vi "Inst_Nexus.vi"(8 "error in":errorcluster, 10 "All Message Queues in":T1, 11 "AjustesPrevios in":refnum<class "AjustesPrevios.lvclass">) -> (0 "error out":errorcluster)   [LabVIEW 2019, in "AjustesPrevios.lvclass"]
uses:
  AjustesPrevios.lvclass
  QMH/Message Queue/All Message Queues.ctl
  QMH/Message Queue/Message Cluster.ctl
  AjustesPrevios.lvclass/AjustesPrevios.ctl
  <vilib>/Utility/error.llb/Error Cluster From Error Code.vi
  QMH/Message Queue/Enqueue Message (Single).vi
  <vilib>/ErrorRing/Error Ring.xnode
  QMH/Message Queue/Message Queue.lvlib
  Instrumento/NEXUS/NEXUS.lvclass
panel:
  out "All States":string[](array[string])
  out "Actual State":string
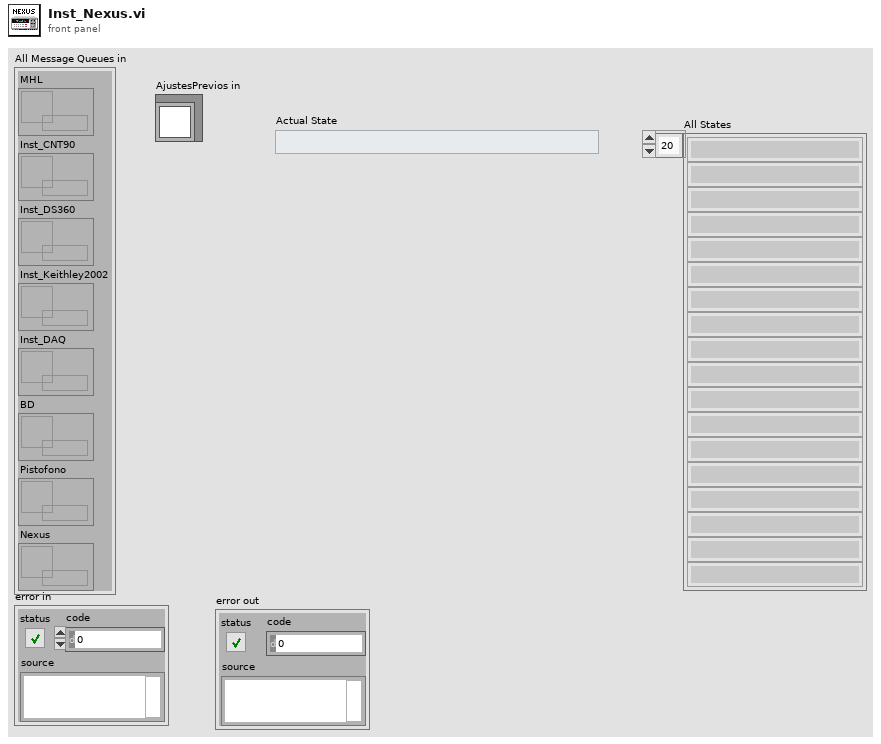
[diagram p1: front panel]
types:
  T1 = typedef "Message Queue.lvlib/All Message Queues.ctl" = cluster{"MHL":refnum<queue>, "Inst_CNT90":refnum<queue>, "Inst_DS360":refnum<queue>, "Inst_Keithley2002":refnum<queue>, "Inst_DAQ":refnum<queue>, "BD":refnum<queue>, "Pistofono":refnum<queue>, "Nexus":refnum<queue>}
  T2 = cluster{"Nivel Emitido Pistófono [dB]":dbl, "Temperatura interna Pistófono[ºC]":dbl, "Presión Medida Pistófono  [hPa]":dbl, "Humedad Relativa Aire [%]":dbl, "FactorCorreccionSensNexus":dbl}
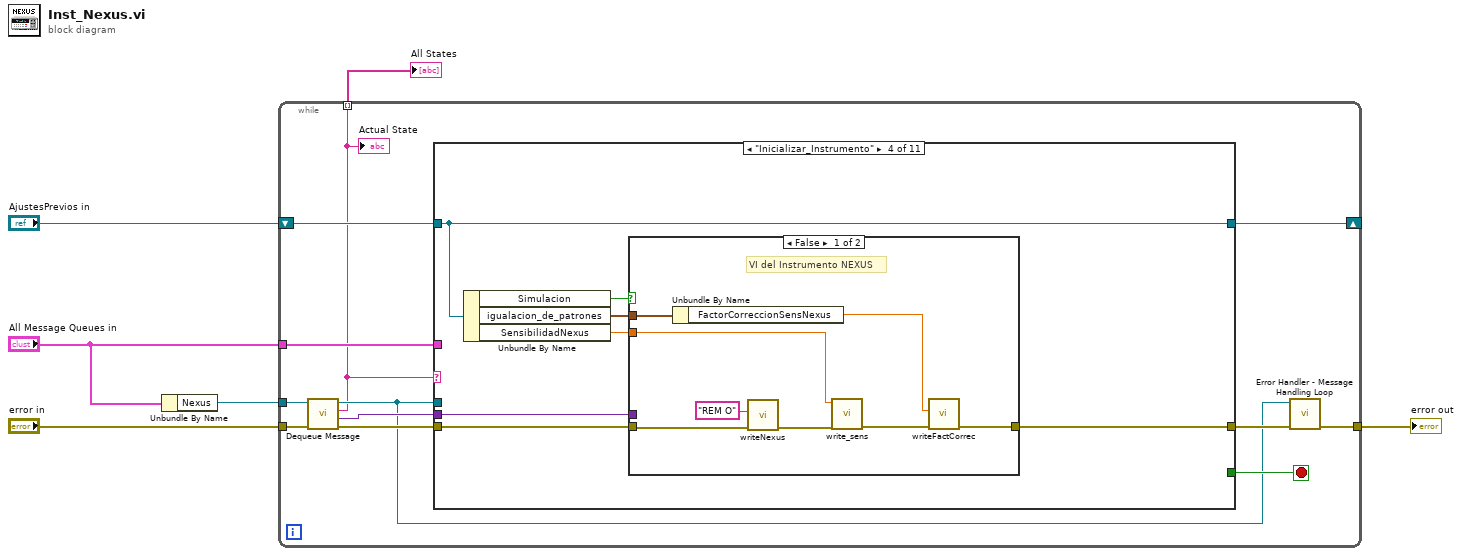
[diagram p0: block diagram]
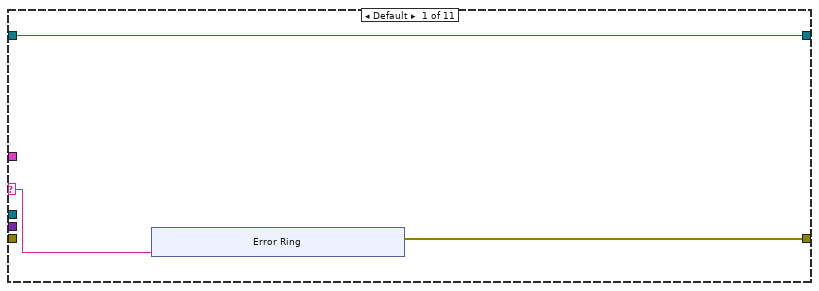
[diagram p2: hidden frame]
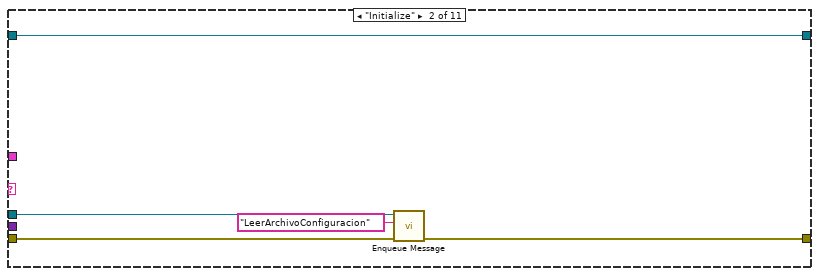
[diagram p3: hidden frame]
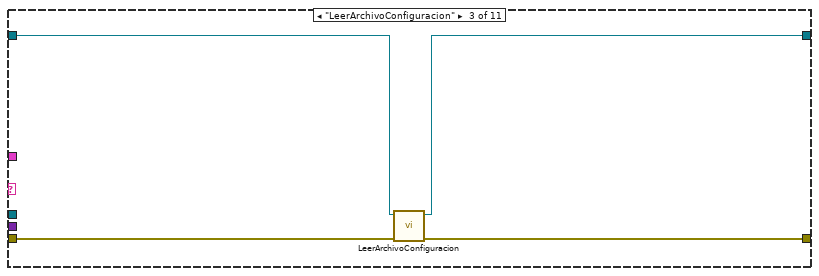
[diagram p4: hidden frame]
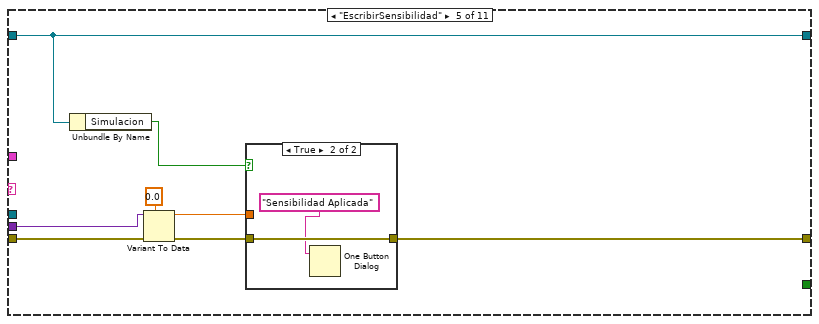
[diagram p6: hidden frame]
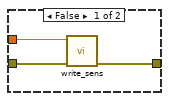
[diagram p7: hidden frame]
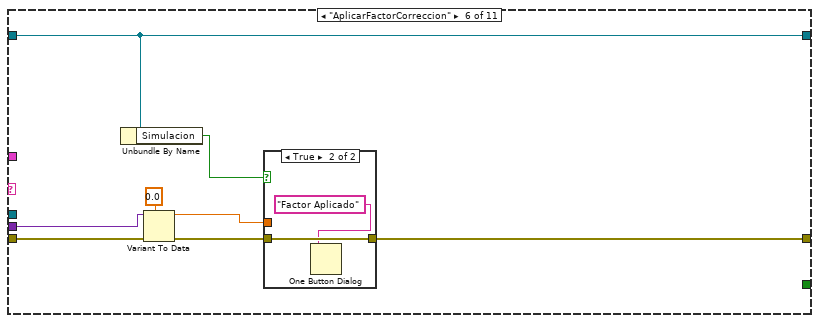
[diagram p8: hidden frame]
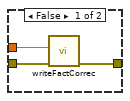
[diagram p9: hidden frame]
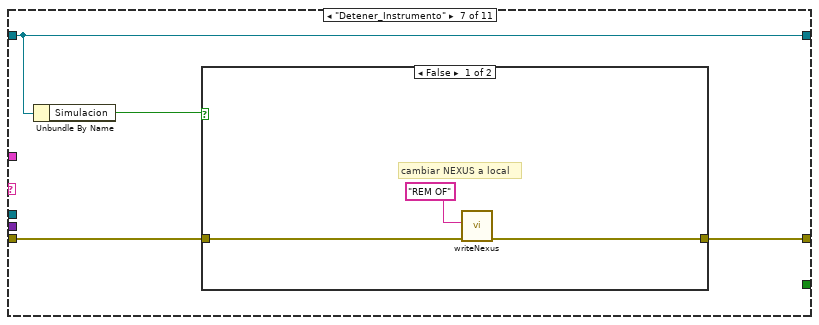
[diagram p10: hidden frame]
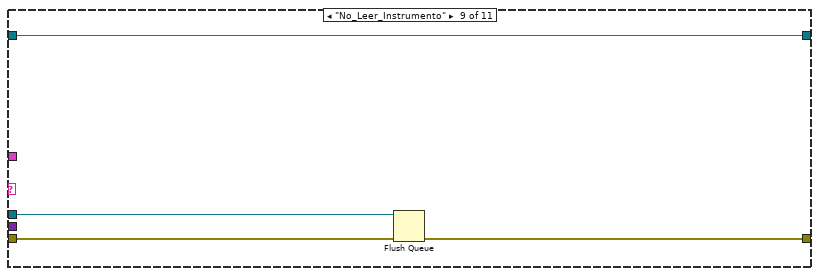
[diagram p13: hidden frame]
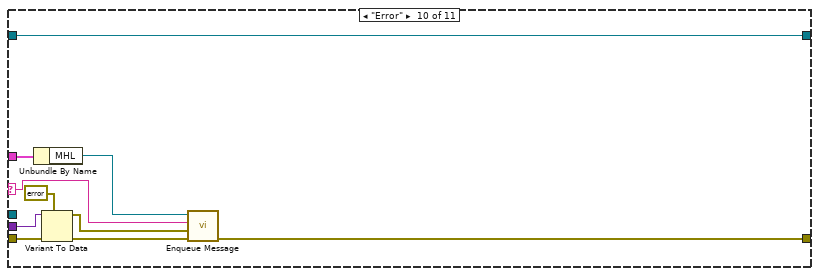
[diagram p14: hidden frame]
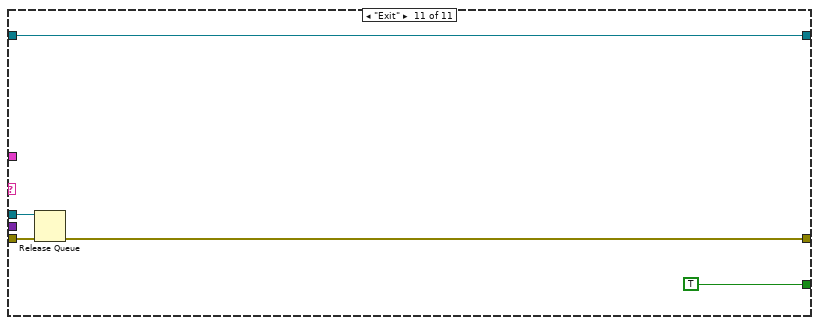
[diagram p15: hidden frame]
diagram:
  n1 = Unbundle By Name("All Message Queues in") -> ("Nexus"=w4:refnum<queue>)
  n2 = while {
    tunnel: "error in" -> [w18]
    tunnel: w4 -> [w17]
    tunnel: "All Message Queues in" -> [w16]
    tunnel: [w9] -> w2
    shift-right: [w12] -> _
    shift-left: "AjustesPrevios in" -> [w15]
    tunnel: [w7] -> w1 mode=indexing
    stop <- w11 stop-if-true
    n3 = call "Dequeue Message.vi"("error in (no error)"=w18, "Message Queue"=w17) -> ("error out"=w13:errorcluster, "Message Data"=w14:variant, "Message"=w7:string, "dup Message Queue"=w8:refnum<queue>)  [unwired: 6 in]
    "Actual State" <- w7
    n4 = case shown="\"Inicializar_Instrumento\"" w7 {
      selector: w7 -> [w21 _ _ _ _ _ _ _ _ w98 _]
      tunnel: w16 -> [_ _ _ _ _ _ _ _ _ w97 _]
      tunnel: w15 -> [w19 w33 w35 w44 w55 w68 w82 w88 w92 w95 w105]
      tunnel: w8 -> [_ w30 _ _ _ _ _ _ w90 _ w107]
      tunnel: w14 -> [_ _ _ w40 w58 w71 _ _ _ w101 _]
      tunnel: w13 -> [_ w32 w37 w43 w61 w74 w80 w89 w93 w102 w108]
      tunnel: [w20 w31 w36 w41 w60 w73 w83 w89 w91 w94 w104] -> w10
      tunnel: [w19 w33 w34 w44 w55 w68 w82 w88 w92 w95 w105] -> w12
      tunnel: [_ _ _ _ _ _ _ _ _ _ TRUE] -> w11
      frame Default {
        n5 = xnode "Error Ring"("parameter 0"=w21) -> ("error out"=w20:errorcluster)
      }
      frame "Initialize" {
        n6 = call-poly "Enqueue Message.vi"("error in (no error)"=w32, "Message"="LeerArchivoConfiguracion", "Message Queue"=w30) -> ("error out"=w31:errorcluster)  [unwired: 7 in, 1 out]
      }
      frame "LeerArchivoConfiguracion" {
        n7 = call "LeerArchivoConfiguracion.vi"("error in"=w37, "AjustesPrevios in"=w35) -> ("error out"=w36:errorcluster, "AjustesPrevios out"=w34:refnum<class "AjustesPrevios.lvclass">)  [unwired: 8 in]
      }
      frame "Inicializar_Instrumento" {
        n8 = Unbundle By Name(w44) -> ("Simulacion"=w42:bool, "igualacion_de_patrones"=w39:T2, "SensibilidadNexus"=w38:dbl)
        n9 = case shown="False" w42 {
          tunnel: [w48 w53] -> w41
          tunnel: w43 -> [w51 w53]
          tunnel: w40 -> [_ _]
          tunnel: w39 -> [w46 _]
          tunnel: w38 -> [w47 _]
          frame False {
            # "VI del Instrumento NEXUS"
            n10 = Unbundle By Name(w46) -> ("FactorCorreccionSensNexus"=w45:dbl)
            n11 = call "writeNexus.vi"("error in (no error)"=w51, "Command"="REM O") -> ("error out"=w50:errorcluster)  [unwired: 8 in, 1 out]
            n12 = call "write_sens.vi"("error in (no error)"=w50, "Sens"=w47) -> ("error out"=w49:errorcluster)  [unwired: 9 in]
            n13 = call "writeFactCorrec.vi"("error in (no error)"=w49, "factor_correccion"=w45) -> ("error out"=w48:errorcluster)  [unwired: 8 in, 1 out]
          }
          frame True {
            # "Simulacion"
          }
        }
      }
      frame "EscribirSensibilidad" {
        n14 = Unbundle By Name(w55) -> ("Simulacion"=w54:bool)
        n15 = Variant To Data(error in=w61, type=0.0, Variant=w58) -> (data=w56:dbl, error out=w59:errorcluster)
        n16 = case shown="True" w54 {
          tunnel: [w64 w66] -> w60
          tunnel: w59 -> [w63 w66]
          tunnel: w56 -> [w62 _]
          frame False {
            n17 = call "write_sens.vi"("error in (no error)"=w63, "Sens"=w62) -> ("error out"=w64:errorcluster)  [unwired: 9 in]
          }
          frame True {
            n18 = One Button Dialog(message="Sensibilidad Aplicada") -> ()  [unwired: 1 in, 1 out]
          }
        }
      }
      frame "AplicarFactorCorreccion" {
        n19 = Unbundle By Name(w68) -> ("Simulacion"=w67:bool)
        n20 = Variant To Data(error in=w74, type=0.0, Variant=w71) -> (data=w69:dbl, error out=w72:errorcluster)
        n21 = case shown="True" w67 {
          tunnel: [w77 w79] -> w73
          tunnel: w72 -> [w76 w79]
          tunnel: w69 -> [w75 _]
          frame False {
            n22 = call "writeFactCorrec.vi"("error in (no error)"=w76, "factor_correccion"=w75) -> ("error out"=w77:errorcluster)  [unwired: 8 in, 1 out]
          }
          frame True {
            n23 = One Button Dialog(message="Factor Aplicado") -> ()  [unwired: 1 in, 1 out]
          }
        }
      }
      frame "Detener_Instrumento" {
        n24 = Unbundle By Name(w82) -> ("Simulacion"=w81:bool)
        n25 = case shown="False" w81 {
          tunnel: [w84 w87] -> w83
          tunnel: w80 -> [w85 w87]
          frame False {
            # "cambiar NEXUS a local"
            n26 = call "writeNexus.vi"("error in (no error)"=w85, "Command"="REM OF") -> ("error out"=w84:errorcluster)  [unwired: 8 in, 1 out]
          }
          frame True {
            # "Simulacion"
          }
        }
      }
      frame "Leer_Instrumento" {
      }
      frame "No_Leer_Instrumento" {
        n27 = Flush Queue(queue=w90, error in (no error)=w93) -> (error out=w91:errorcluster)  [unwired: 2 out]
      }
      frame "Error" {
        n28 = Unbundle By Name(w97) -> ("MHL"=w96:refnum<queue>)
        n29 = Variant To Data(error in=w102, type=errorcluster {"status"=FALSE, "code"=0, "source"=""} ("error constant"), Variant=w101) -> (data=w99:errorcluster, error out=w100:errorcluster)
        n30 = call-poly "Enqueue Message.vi"("error in (no error)"=w100, "Message Data"=w99, "Message"=w98, "Message Queue"=w96) -> ("error out"=w94:errorcluster)  [unwired: 6 in, 1 out]
      }
      frame "Exit" {
        n31 = Release Queue(queue=w107, error in (no error)=w108) -> (error out=w104:errorcluster)  [unwired: 1 in, 2 out]
      }
    }
    n32 = call "Error Handler - Message Handling Loop.vi"("error in (no error)"=w10, "Message Queue"=w8) -> ("dup error in"=w9:errorcluster)  [unwired: 8 in, 1 out]
  }
  "error out" <- w2
  "All States" <- w1
